vi "Initialize.vi"(8 "error in (no error)":errorcluster, 9 "Reset (True)":bool=TRUE, 10 "ID Query (True)":bool=TRUE, 11 "VISA resource name":refnum<visa-resource-name>) -> (0 "error out":errorcluster, 3 "VISA resource name out":refnum<visa-resource-name>)   [LabVIEW 2023, in "RIGOL DS1054Z Driver.lvlib"]
doc: "Establishes communication with the instrument and optionally performs an instrument identification query and/or an instrument reset. It also places the instrument in a default state needed for other instrument driver operations. Therefore, call this VI before calling other instrument driver VIs for this instrument. Generally, you need to call the Initialize VI only once at the beginning of an application."
uses:
  <instrlib>/RIGOL-DS1054Z-LabVIEW/RIGOL DS1054Z Driver.lvlib
panel:
  # "(c) 2010-2012, RIGOL Technologies, Inc.  All Rights Reserved."
  # "Reset can be set to true only if the firmware version is 00.03.01.00.00 or later."
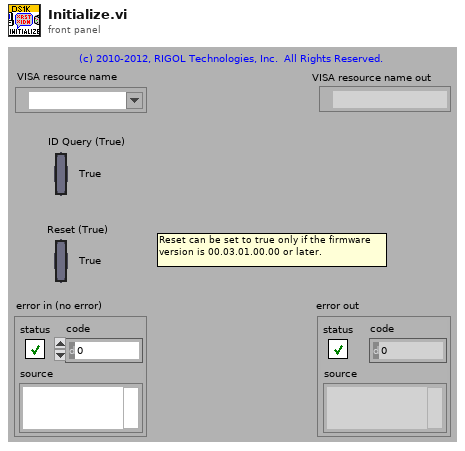
[diagram p1: front panel]
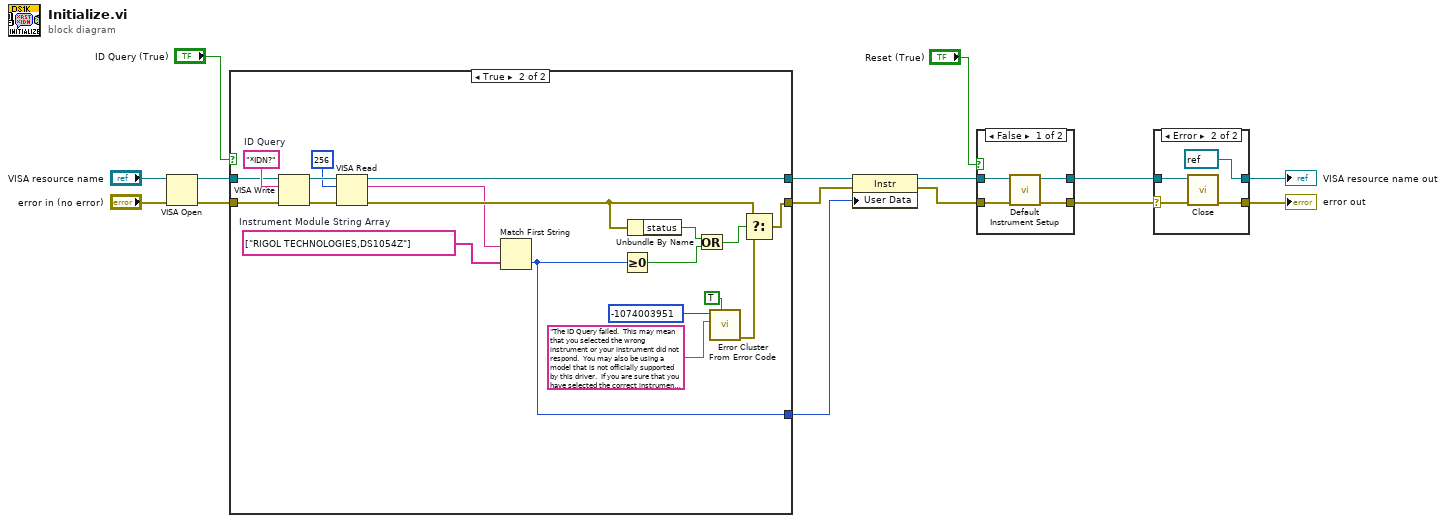
[diagram p0: block diagram]
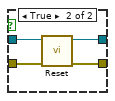
[diagram p3: hidden frame]
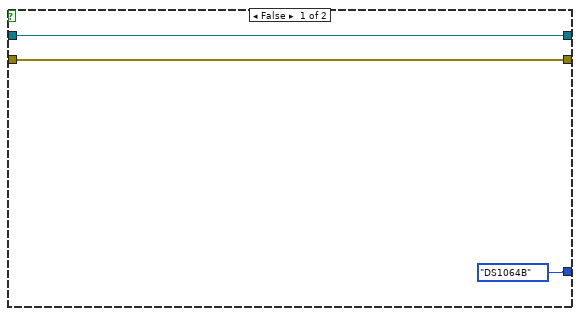
[diagram p4: hidden frame]
diagram:
  n1 = VISA Open(error in (no error)="error in (no error)", VISA resource name="VISA resource name") -> (VISA resource name=w3:refnum<visa-resource-name>, error out=w2:errorcluster)  [unwired: 3 out]
  n2 = case shown="True" "ID Query (True)" {
    tunnel: [w18 w37] -> w6
    tunnel: [w17 w35] -> w8
    tunnel: w2 -> [w18 w36]
    tunnel: w3 -> [w17 w22]
    tunnel: [enum16{"DS1064B"}."DS1064B" ("Instrument Module") w21] -> w4
    frame False {
    }
    frame True {
      w20 = string[] ["RIGOL TECHNOLOGIES,DS1054Z"]  # Instrument Module String Array
      w31 = "*IDN?"  # ID Query
      n3 = VISA Write(VISA resource name=w22, write buffer=w31, error in (no error)=w36) -> (VISA resource name out=w34:refnum<visa-resource-name>, error out=w33:errorcluster)  [unwired: 1 out]
      n4 = VISA Read(VISA resource name=w34, byte count=u32 256, error in (no error)=w33) -> (VISA resource name out=w35:refnum<visa-resource-name>, read buffer=w19:string, error out=w26:errorcluster)  [unwired: 1 out]
      n5 = Match First String(2:w20, 3:w19) -> (0:w21:i32)  [unwired: 1 out]
      n6 = Greater Or Equal To 0?(x=w21) -> (x >= 0?=w24:bool)
      n7 = Unbundle By Name(w26) -> ("status"=w25:bool)
      n8 = Or(x=w25, y=w24) -> (x .or. y?=w23:bool)
      n9 = call <vilib>:"Error Cluster From Error Code.vi"("show call chain? (False)"=TRUE, "error message (\"\")"="The ID Query failed.  This may mean that you selected the wrong instrument or your instrument did not respond.  You may also be using a model that is not officially supported by this driver.  If you are sure that you have selected the correct instrument and it is responding, try disabling the ID Query." ("Source (VI Name)"), "error code (0)"=-1074003951 ("Code")) -> ("error out"=w30:errorcluster)  [unwired: 1 in, 5 out]
      n10 = Select(t=w26, s=w23, f=w30) -> (s? t:f=w37:errorcluster)
    }
  }
  n11 = property class="Instr"(reference=w8, error in=w6, "User Data"=w4) -> (reference out=w7:refnum<visa-resource-name>, error out=w5:errorcluster)
  n12 = case shown="False" "Reset (True)" {
    tunnel: w5 -> [w40 w42]
    tunnel: [w38 w45] -> w9
    tunnel: w7 -> [w41 w43]
    tunnel: [w39 w44] -> w10
    frame False {
      n13 = call <instrlib>:"Default Instrument Setup.vi"("error in (no error)"=w40, "VISA resource name"=w41) -> ("error out"=w38:errorcluster, "VISA resource name out"=w39:refnum<visa-resource-name>)  [unwired: 8 out]
    }
    frame True {
      n14 = call <instrlib>:"Reset.vi"("error in (no error)"=w42, "VISA resource name"=w43) -> ("error out"=w45:errorcluster, "VISA resource name out"=w44:refnum<visa-resource-name>)  [unwired: 8 out]
    }
  }
  n15 = case shown="Error" w9 {
    selector: w9 -> [w46 w49]
    tunnel: w10 -> [w47 w50]
    tunnel: [w47 refnum<visa-resource-name> refnum ("VISA resource name out")] -> w1
    tunnel: [w46 w51] -> w11
    frame No Error {
    }
    frame Error {
      n16 = call <instrlib>:"Close.vi"("error in (no error)"=w49, "VISA resource name"=w50) -> ("error out"=w51:errorcluster)  [unwired: 9 out]
    }
  }
  "VISA resource name out" <- w1
  "error out" <- w11
